vi "AlliGator Square Gated IRF Fit Cursors String.vi"(8 "Error In":errorcluster, 9 "Cursor Positions Array":dbl[](array[numeric]), 11 "Cursor Names Array":string[](array[string])) -> (0 "Error Out":errorcluster, 2 "Message":string)   [LabVIEW 2021, in "AlliGator IRF.lvlib"]
doc: "Creates string describing the boundaries between regions in a square gate."
uses:
  AlliGator IRF.lvlib
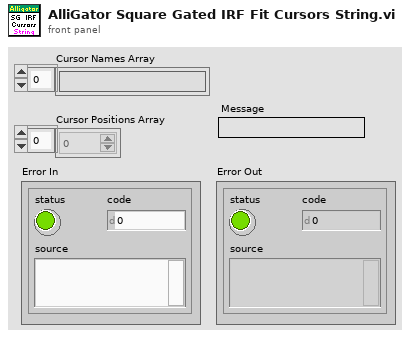
[diagram p1: front panel]
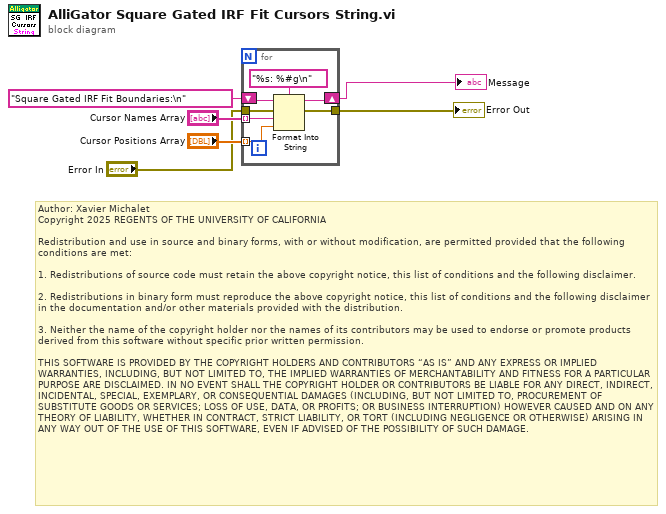
[diagram p0: block diagram]
diagram:
  # "Author: Xavier Michalet\nCopyright 2025 REGENTS OF THE UNIVERSITY OF CALIFORNIA\n\nRedistribution and use in source and binary forms, with or without modification, are permitted provided that the following conditions are met:\n\n1. Redistributions of source code must retain the above copyright notice, this list of conditions and the following disclaimer.\n\n2. Redistributions in binary form must reproduce the above copyright notice, this list of conditions and the following disclaimer in the documentation and/or other materials provided with the distribution.\n\n3. Neither the name of the copyright holder nor the names of its contributors may be used to endorse or promote products derived from this software without specific prior written permission.\n\nTHIS SOFTWARE IS PROVIDED BY THE COPYRIGHT HOLDERS AND CONTRIBUTORS “AS IS” AND ANY EXPRESS OR IMPLIED WARRANTIES, INCLUDING, BUT NOT LIMITED TO, THE IMPLIED WARRANTIES OF MERCHANTABILITY AND FITNESS FOR A PARTICULAR PURPOSE ARE DISCLAIMED. IN NO EVENT SHALL THE COPYRIGHT HOLDER OR CONTRIBUTORS BE LIABLE FOR ANY DIRECT, INDIRECT, INCIDENTAL, SPECIAL, EXEMPLARY, OR CONSEQUENTIAL DAMAGES (INCLUDING, BUT NOT LIMITED TO, PROCUREMENT OF SUBSTITUTE GOODS OR SERVICES; LOSS OF USE, DATA, OR PROFITS; OR BUSINESS INTERRUPTION) HOWEVER CAUSED AND ON ANY THEORY OF LIABILITY, WHETHER IN CONTRACT, STRICT LIABILITY, OR TORT (INCLUDING NEGLIGENCE OR OTHERWISE) ARISING IN ANY WAY OUT OF THE USE OF THIS SOFTWARE, EVEN IF ADVISED OF THE POSSIBILITY OF SUCH DAMAGE."
  n1 = for {
    tunnel: "Cursor Names Array" -> [w13] mode=indexing
    tunnel: "Cursor Positions Array" -> [w12] mode=indexing
    shift-right: [w10] -> w1
    shift-left: "Square Gated IRF Fit Boundaries:\n" -> [w11]
    tunnel: "Error In" -> [w8]
    tunnel: [w7] -> w2
    n2 = Format Into String(format string="%s: %#g\n", initial string=w11, error in=w8, w13, w12) -> (resulting string=w10:string, error out=w7:errorcluster)
  }
  "Error Out" <- w2
  "Message" <- w1
